vi "GetG.vi"(0 "q":dbl[](array[numeric]), 7 "m":dbl, 9 "L":dbl, 11 "L1":dbl) -> (8 "C":T1)   [LabVIEW 2019]
uses:
  <vilib>/Analysis/Matrix/Datatypes/RealMatrix.ctl
  <vilib>/Analysis/Matrix/NI_Matrix.lvlib
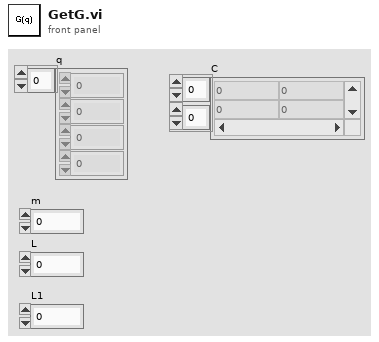
[diagram p1: front panel]
types:
  T1 = typedef "NI_Matrix.lvlib/RealMatrix.ctl" = dbl[][]
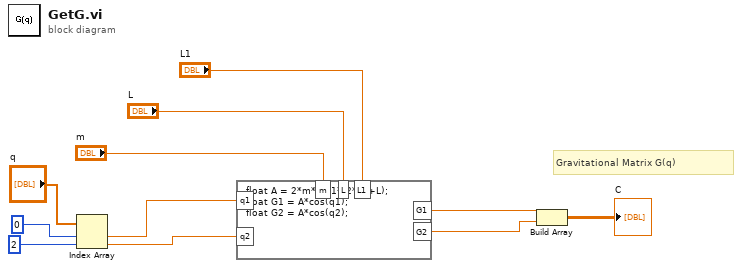
[diagram p0: block diagram]
diagram:
  # "Gravitational Matrix G(q)"
  n1 = Index Array(array="q", index #1=0 ("index (row)"), index #2=2 ("index (col)")) -> (element #1=w3:dbl, element #2=w2:dbl)
  n2 = formula code="float A = 2*m*9.81*(2*L1+L);\nfloat G1 = A*cos(q1);\nfloat G2 = A*cos(q2);"("m"="m", "L"="L", "L1"="L1", "q1"=w3, "q2"=w2) -> ("G1"=w5:dbl, "G2"=w4:dbl)
  n3 = Build Array(w5, w4) -> (→"C":T1)
